vi "Read Label.vi"(8 "error in (no error)":errorcluster, 11 "Message":refnum<class "MSG.lvclass">) -> (0 "error out":errorcluster, 2 "Label":string caption="Label (or Message Class)", 3 "Message":refnum<class "MSG.lvclass">)   [LabVIEW 2011, in "Messenging.lvlib" / "MSG.lvclass"]
uses:
  MSG.lvclass
panel:
  # "Uses Message Class Name if Label is empty"
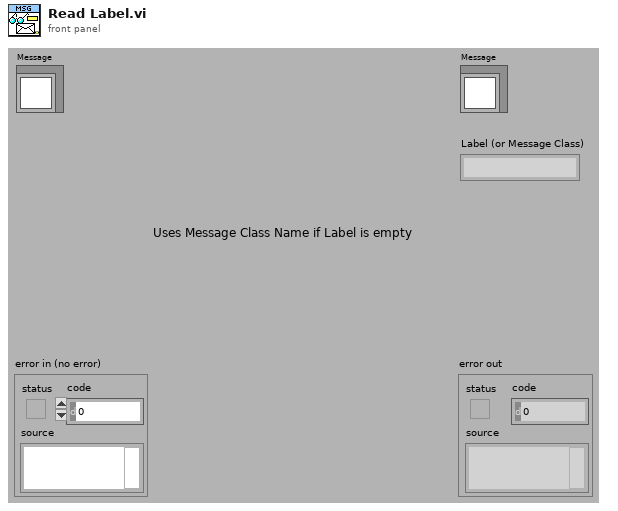
[diagram p1: front panel]
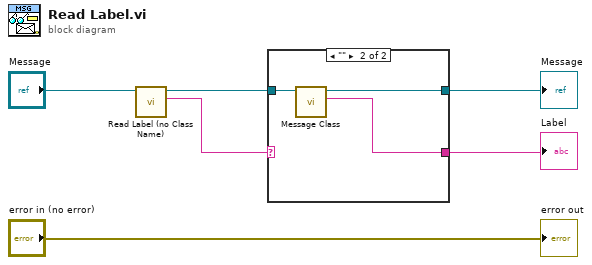
[diagram p0: block diagram]
diagram:
  n1 = call "Read Label (no Class Name).vi"("MSG.lvclass in"="Message") -> ("Label"=w1:string, "MSG.lvclass out"=w2:refnum<class "MSG.lvclass">)  [unwired: 9 out]
  n2 = case shown="\"\"" w1 {
    selector: w1 -> [w7 _]
    tunnel: w2 -> [w8 w11]
    tunnel: [w8 w10] -> w5
    tunnel: [w7 w9] -> w4
    frame "False", Default {
    }
    frame "" {
      n3 = call-dynamic "Message Class.vi"("Message"=w11) -> ("Message Class"=w9:string, "Message"=w10:refnum<class "MSG.lvclass">)  [unwired: 1 in, 8 out]
    }
  }
  "Message" <- w5
  "Label" <- w4
  "error out" <- "error in (no error)"
